vi "test Galvo.vi"   [LabVIEW 2012]
uses:
  Galvo.lvclass
  <vilib>/Distrio/Murmex/Murmex/Murmex.lvclass
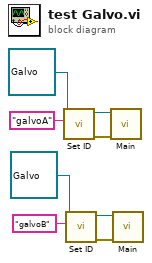
[diagram p0: block diagram]
diagram:
  n1 = call <vilib>:"Set ID.vi"("id"="galvoA", "Murmex in"=refnum<class "Galvo.lvclass"> refnum ("Galvo.lvclass")) -> ("error out"=w6:errorcluster, "Murmex out"=w7:refnum<class "Galvo.lvclass">)  [unwired: 8 in]
  n2 = call <vilib>:"Set ID.vi"("id"="galvoB", "Murmex in"=refnum<class "Galvo.lvclass"> refnum ("Galvo.lvclass")) -> ("error out"=w3:errorcluster, "Murmex out"=w2:refnum<class "Galvo.lvclass">)  [unwired: 8 in]
  n3 = call-dynamic "Main.vi"("error in (no error)"=w6, "GalvoBase in"=w7) -> ()  [unwired: 8 in, 2 out]
  n4 = call-dynamic "Main.vi"("error in (no error)"=w3, "GalvoBase in"=w2) -> ()  [unwired: 8 in, 2 out]
